vi "Actor Core.vi"(8 "error in":errorcluster, 11 "IED in":refnum<class "IED.lvclass">) -> (0 "error out":errorcluster, 3 "Actor out":refnum<class "Actor.lvclass">)   [LabVIEW 2018, in "IED Actor.lvlib" / "IED.lvclass"]
doc: "(<B>Filename</B>: Actor Framework.lvlib:Actor.lvclass:Actor Core.vi)\n\nReceives messages to the actor, reacts to them, and initiates any error handling that may shut the actor down.\n\nDescendant classes may override this VI to append parallel tasks for the actor to complete while it handles messages. Overrides use the Call Parent Method node."
uses:
  IED.lvclass
  C:/Users/Administrator/Desktop/2018LabVIEW EMS/EMS Generic Actor/EMS Generic/EMS Generic.lvclass
  <vilib>/ActorFramework/Actor/Actor.lvclass
  EMS Generic Actor/EMS Generic/EMS Generic.lvclass/EMS Generic.ctl
  IED.lvclass/IED.ctl
  <vilib>/ORNL/CSEISMIC DDS/CSEISMIC DDS Base/CSEISMIC DDS.lvclass/CSEISMIC DDS.ctl
  <vilib>/ORNL/CSEISMIC DDS/CSEISMIC DDS Base/Data Types/Controls/Timestamp.ctl
  <vilib>/ORNL/CSEISMIC DDS/CSEISMIC DDS Base/Accessors/Write DDS Reference.vi
  <vilib>/ORNL/CSEISMIC DDS/CSEISMIC DDS Base/Accessors/Read DDS Reference.vi
  <vilib>/ORNL/CSEISMIC DDS/DDS Reader/DDS Reader.lvclass
  C:/Program Files (x86)/National Instruments/LabVIEW 2018/vi.lib/ORNL/CSEISMIC DDS/CSEISMIC DDS Base/CSEISMIC DDS.lvclass
  <vilib>/ORNL/CSEISMIC DDS/CSEISMIC DDS Base/Error Handler.vi
  Device DDS Communications Framework/Device DDS Communications/Device DDS Communications.lvclass
  <vilib>/ORNL/CSEISMIC DDS/CSEISMIC DDS Base/CSEISMIC DDS.lvclass
  EMS Generic Actor/EMS Generic/EMS Generic.lvclass
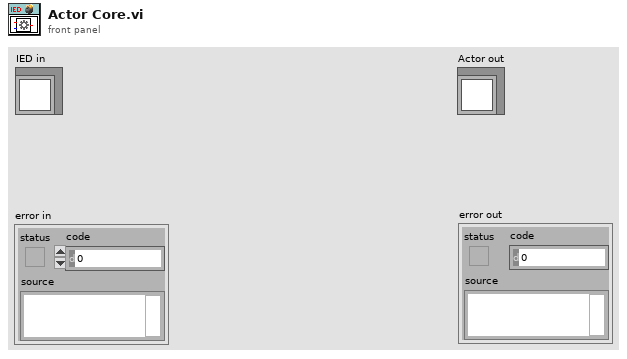
[diagram p1: front panel]
types:
  T1 = typedef "CSEISMIC DDS.lvlib/CSEISMIC DDS.lvclass/Timestamp.ctl" = cluster{"Seconds":u64, "Remainder":u64}
  T2 = typedef "CSEISMIC DDS.lvlib/CSEISMIC DDS.lvclass/DeviceID.ctl" = string
  T3 = typedef "CSEISMIC DDS.lvlib/CSEISMIC DDS.lvclass/IED_Status.ctl" = cluster{"DeviceID":T2, "Timestamp":T1, "MicrogridID":u8, "Active":bool, "Inactive":bool, "Error":i32, "Fault":bool, "ErrorString":string}
  T4 = typedef "LVDDS_library.lvlib/DDS Sample Info.ctl" = cluster{"DDS_SampleStateKind":enum32{"DDS_INVALID_SAMPLE_STATE", "DDS_READ_SAMPLE_STATE", "DDS_NOT_READ_SAMPLE_STATE"}, "DDS_ViewStateKind":enum32{"DDS_INVALID_SAMPLE_STATE", "DDS_NEW_VIEW_STATE", "DDS_NOT_NEW_VIEW_STATE"}, "DDS_InstanceStateKind":enum32{"DDS_INVALID_STATE", "DDS_ALIVE_INSTANCE_STATE", "DDS_NOT_ALIVE_DISPOSED_INSTANCE_STATE", "", "DDS_NOT_ALIVE_NO_WRITERS_INSTANCE_STATE"}, "sec":i32, "nanosec":u32, "valid_data":bool}
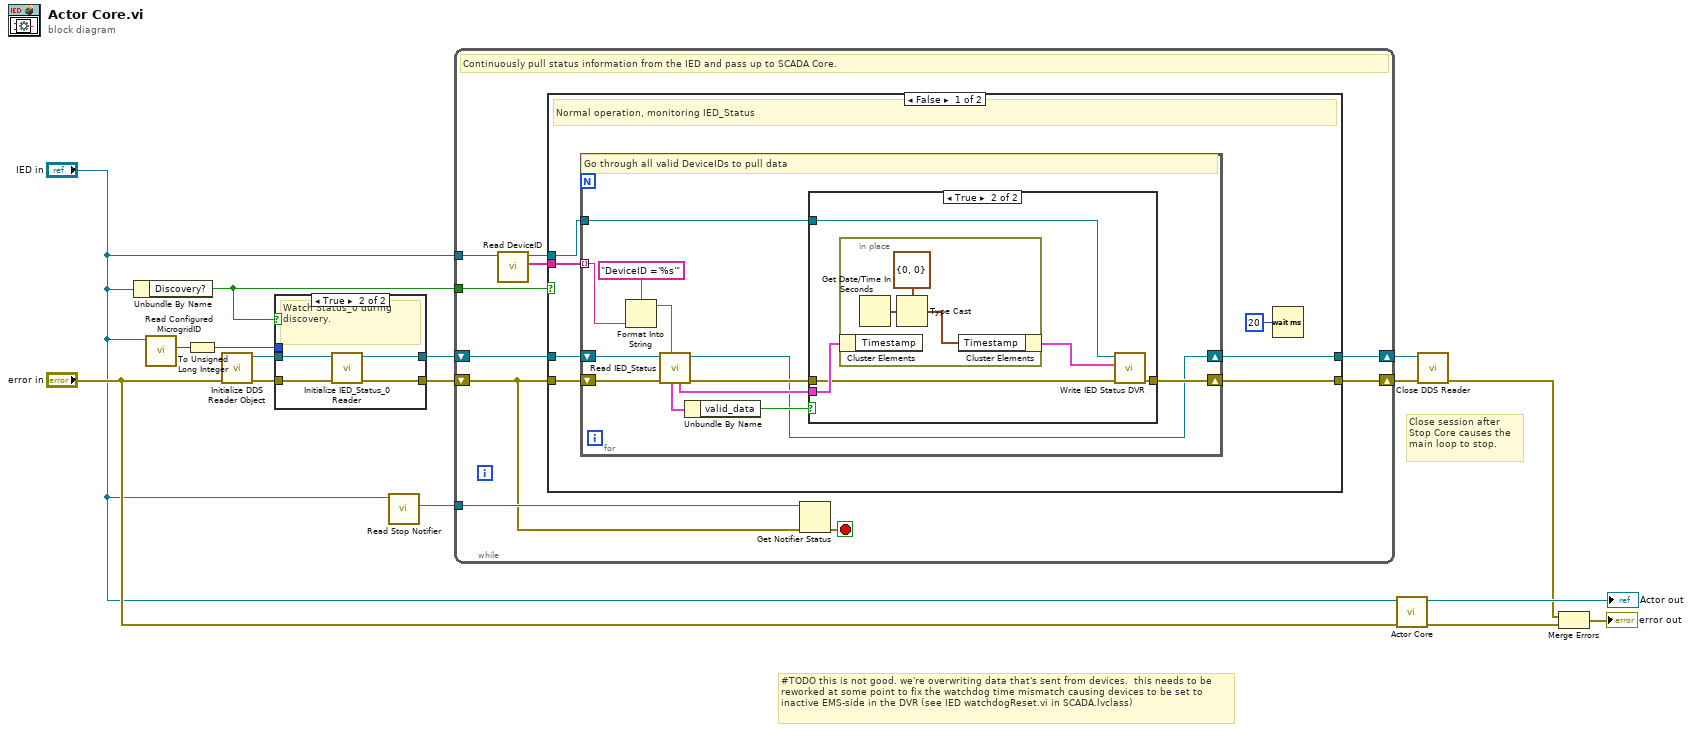
[diagram p0: block diagram]
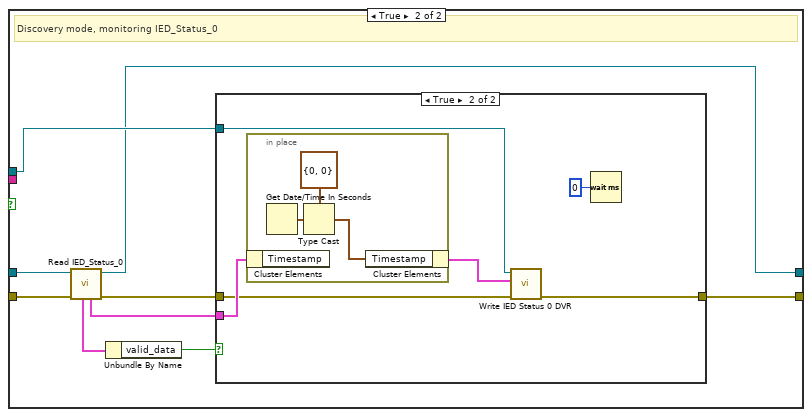
[diagram p3: hidden frame]
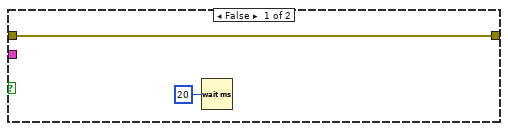
[diagram p4: hidden frame]
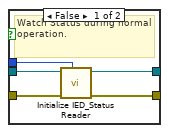
[diagram p5: hidden frame]
diagram:
  # "#TODO this is not good. we're overwriting data that's sent from devices.  this needs to be reworked at some point to fix the watchdog time mismatch causing devices to be set to inactive EMS-side in the DVR (see IED watchdogReset.vi in SCADA.lvclass)"
  # "Close session after Stop Core causes the main loop to stop."
  n1 = Unbundle By Name("IED in") -> ("Discovery?"=w1:bool)
  n2 = call "Read Configured MicrogridID.vi"("EMS Generic in"="IED in") -> ("Microgrid ID"=w14:u8)  [unwired: 8 in, 2 out]
  n3 = To Unsigned Long Integer(number=w14) -> (unsigned 32bit integer=w9:u32)
  n4 = call <vilib>:"Initialize DDS Reader Object.vi"("error in"="error in") -> ("error out"=w10:errorcluster, "DDS Reader out"=w11:refnum<class "DDS Reader.lvclass">)  [unwired: 9 in]
  n5 = case shown="True" w1 {
    tunnel: w11 -> [w21 w25]
    tunnel: w10 -> [w20 w22]
    tunnel: w9 -> [w19 _]
    tunnel: [w18 w24] -> w8
    tunnel: [w17 w23] -> w7
    frame False {
      # "Watch Status during normal operation."
      n6 = call <vilib>:"Initialize IED_Status Reader.vi"("MicrogridID"=w19, "error in"=w20, "DDS Reader in"=w21) -> ("error out"=w17:errorcluster, "DDS Reader out"=w18:refnum<class "DDS Reader.lvclass">)  [unwired: 7 in]
    }
    frame True {
      # "Watch Status_0 during discovery."
      n7 = call <vilib>:"Initialize IED_Status_0 Reader.vi"("error in"=w22, "DDS Reader in"=w25) -> ("error out"=w23:errorcluster, "DDS Reader out"=w24:refnum<class "DDS Reader.lvclass">)  [unwired: 8 in]
    }
  }
  n8 = call "Read Stop Notifier.vi"("EMS Generic in"="IED in") -> ("stop"=w13:refnum<notifier>)  [unwired: 9 in, 1 out]
  n9 = while {
    tunnel: w13 -> [w35]
    shift-right: [w27] -> w5
    shift-left: w7 -> [w29]
    tunnel: w1 -> [w32]
    tunnel: "IED in" -> [w33]
    shift-right: [w28] -> w6
    shift-left: w8 -> [w30]
    stop <- w34 stop-if-true
    # "Continuously pull status information from the IED and pass up to SCADA Core."
    n10 = call-dynamic "Read DeviceID.vi"("Device DDS Communications in"=w33) -> ("DeviceID"=w31:T2[], "Device DDS Communications out"=w26:refnum<class "IED.lvclass">)  [unwired: 9 in]
    n11 = case shown="False" w32 {
      tunnel: w31 -> [w41 _]
      tunnel: w30 -> [w42 w72]
      tunnel: w29 -> [w40 w71]
      tunnel: [w39 w64] -> w28
      tunnel: [w38 w66] -> w27
      tunnel: w26 -> [w37 w65]
      frame False {
        # "Normal operation, monitoring IED_Status"
        n12 = for {
          shift-right: [w43] -> w39
          shift-left: w42 -> [w54]
          shift-right: [w45] -> w38
          shift-left: w40 -> [w53]
          tunnel: w41 -> [w51] mode=indexing
          tunnel: w37 -> [w46]
          # "Go through all valid DeviceIDs to pull data"
          n13 = Format Into String(format string="DeviceID ='%s'", w51) -> (resulting string=w50:string)  [unwired: 2 in, 1 out]
          n14 = call <vilib>:"Read IED_Status.vi"("Query condition"=w50, "error in"=w53, "DDS Reader in"=w54) -> ("error out"=w48:errorcluster, "DDS Reader out"=w43:refnum<class "DDS Reader.lvclass">, "data"=w47:T3, "DDS Sample Info"=w49:T4)  [unwired: 5 in]
          n15 = Unbundle By Name(w49) -> ("valid_data"=w44:bool)
          n16 = case shown="True" w44 {
            tunnel: w47 -> [_ w60]
            tunnel: w48 -> [w55 w59]
            tunnel: [w55 w58] -> w45
            tunnel: w46 -> [_ w57]
            frame False {
            }
            frame True {
              n17 = in-place {
                n18 = in-place-cluster #1(w60) -> ()  [unwired: 1 out]
                n19 = Get Date/Time In Seconds() -> (seconds since 1Jan1904=w62:timestamp)
                n20 = Type Cast(type=T1 {"Seconds"=0, "Remainder"=0} ("Timestamp"), x=w62) -> (*(type *) &x=w61:T1)
                n21 = in-place-cluster #1("Timestamp"=w61) -> (w56:T3)
              }
              n22 = call "Write IED Status DVR.vi"("error in"=w59, "IED_Status"=w56, "SCADA in"=w57) -> ("error out"=w58:errorcluster)  [unwired: 7 in, 1 out]
            }
          }
        }
        n23 = Wait (ms)(milliseconds to wait=u32 20) -> ()  [unwired: 1 out]
      }
      frame True {
        # "Discovery mode, monitoring IED_Status_0"
        n24 = call <vilib>:"Read IED_Status_0.vi"("error in"=w71, "DDS Reader in"=w72) -> ("error out"=w67:errorcluster, "DDS Reader out"=w64:refnum<class "DDS Reader.lvclass">, "data"=w68:T3, "DDS Sample Info"=w70:T4)  [unwired: 6 in]
        n25 = Unbundle By Name(w70) -> ("valid_data"=w69:bool)
        n26 = case shown="True" w69 {
          tunnel: w68 -> [_ w79]
          tunnel: w67 -> [w73 w77]
          tunnel: [w73 w76] -> w66
          tunnel: w65 -> [_ w75]
          frame False {
            n27 = Wait (ms)(milliseconds to wait=u32 20) -> ()  [unwired: 1 out]
          }
          frame True {
            n28 = in-place {
              n29 = in-place-cluster #2(w79) -> ()  [unwired: 1 out]
              n30 = Get Date/Time In Seconds() -> (seconds since 1Jan1904=w82:timestamp)
              n31 = Type Cast(type=T1 {"Seconds"=0, "Remainder"=0} ("Timestamp"), x=w82) -> (*(type *) &x=w81:T1)
              n32 = in-place-cluster #2("Timestamp"=w81) -> (w78:T3)
            }
            n33 = call "Write IED Status 0 DVR.vi"("error in"=w77, "IED_Status_0"=w78, "EMS Generic in"=w75) -> ("error out"=w76:errorcluster)  [unwired: 7 in, 1 out]
            n34 = Wait (ms)(milliseconds to wait=u32 0) -> ()  [unwired: 1 out]
          }
        }
      }
    }
    n35 = Get Notifier Status(notifier=w35, error in (no error)=w29) -> (error out=w34:errorcluster)  [unwired: 4 out]
  }
  n36 = call-parent "Actor Core.vi"("error in"="error in", "Actor in"="IED in") -> ("error out"=w15:errorcluster, "Actor out"=→"Actor out":refnum<class "Actor.lvclass">)  [unwired: 8 in]
  n37 = call <vilib>:"Close DDS Reader.vi"("error in"=w5, "DDS Reader in"=w6) -> ("error out"=w2:errorcluster)  [unwired: 9 in]
  n38 = Merge Errors(w2, w15) -> (→"error out":errorcluster)
